vi "Open.vi"(8 "error in (no error)":errorcluster, 11 "MelsecTCP in":refnum<class "InovanceModbusTcp.lvclass">) -> (0 "error out":errorcluster, 3 "MelsecTCP out":refnum<class "InovanceModbusTcp.lvclass">)   [LabVIEW 2020, in "HslCommunication.lvlib" / "InovanceModbusTcp.lvclass"]
uses:
  InovanceModbusTcp.lvclass
  InovanceModbusTcp.lvclass/InovanceModbusTcp.ctl
  E:/Git/Libraries/develop/HslCommunication/_Dependenciecs/HslCommunication.dll
  _Dependenciecs/HslCommunication.dll
  Read series.vi
  Read ipAddress.vi
  Read port.vi
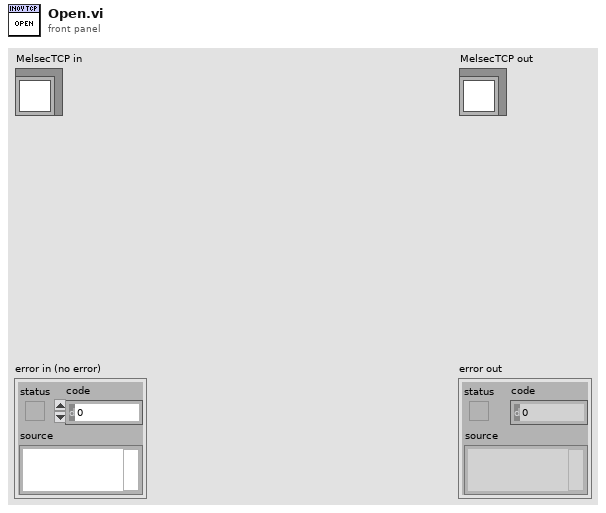
[diagram p1: front panel]
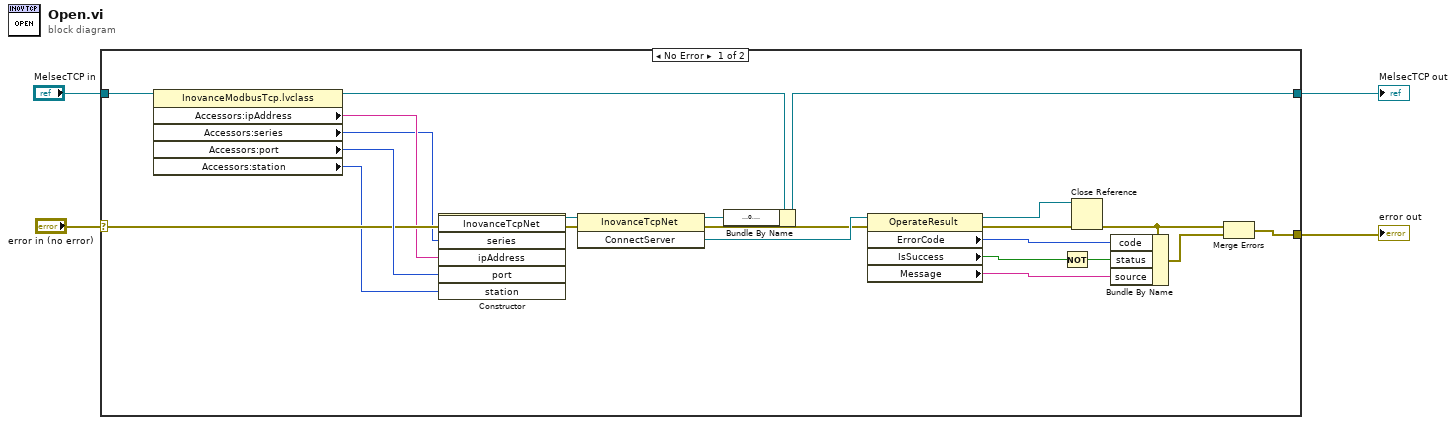
[diagram p0: block diagram]
diagram:
  n1 = case shown="No Error" "error in (no error)" {
    selector: "error in (no error)" -> [w8 w28]
    tunnel: "MelsecTCP in" -> [w26 w27]
    tunnel: [w25 w27] -> w1
    tunnel: [w19 w28] -> w2
    frame No Error {
      n2 = property class="InovanceModbusTcp.lvclass"(reference=w26) -> (reference out=w10:refnum<class "InovanceModbusTcp.lvclass">, "Accessors:ipAddress"=w7:string, "Accessors:series"=w5:i32, "Accessors:port"=w9:i32, "Accessors:station"=w6:u8)  [unwired: 1 in, 1 out]
      n3 = constructor class="InovanceTcpNet"(error in=w8, "series"=w5, "ipAddress"=w7, "port"=w9, "station"=w6) -> (reference out=w14:refnum<k24>, error out=w13:errorcluster)  [unwired: 2 in, 5 out]
      n4 = invoke class="InovanceTcpNet" method="ConnectServer"(reference=w14, error in=w13) -> (reference out=w11:refnum<k24>, error out=w16:errorcluster, "ConnectServer"=w18:refnum<k24>)  [unwired: 1 in]
      n5 = Bundle By Name(cluster=w10, "reference"=w11) -> (w25:refnum<class "InovanceModbusTcp.lvclass">)
      n6 = property class="OperateResult"(reference=w18, error in=w16) -> (reference out=w17:refnum<k24>, error out=w15:errorcluster, "ErrorCode"=w22:i32, "IsSuccess"=w12:bool, "Message"=w20:string)
      n7 = Not(x=w12) -> (.not. x?=w21:bool)
      n8 = Close Reference(reference=w17, error in (no error)=w15) -> (error out=w23:errorcluster)
      n9 = Bundle By Name(cluster=w23, "code"=w22, "status"=w21, "source"=w20) -> (w24:errorcluster)
      n10 = Merge Errors(w23, w24) -> (w19:errorcluster)
    }
    frame Error {
    }
  }
  "error out" <- w2
  "MelsecTCP out" <- w1
